vi "Ejercicio 2.4.vi"() -> ()   [LabVIEW 2013]
panel:
  in  "Funcion":T1(ring)
  in  "stop 2":bool
  out "Waveform Graph":dbl[](graph)
  in  "Amplitud":dbl
  in  "Frecuencia":dbl
  in  "Cantidad de muestras":i32=20
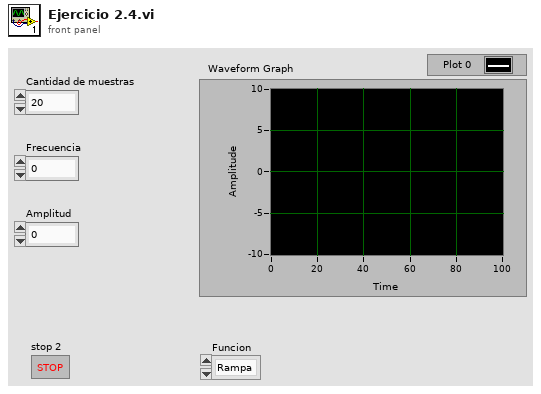
[diagram p1: front panel]
types:
  T1 = enum16{"Rampa", "Seno", "Triangular", "Cuadrado"}
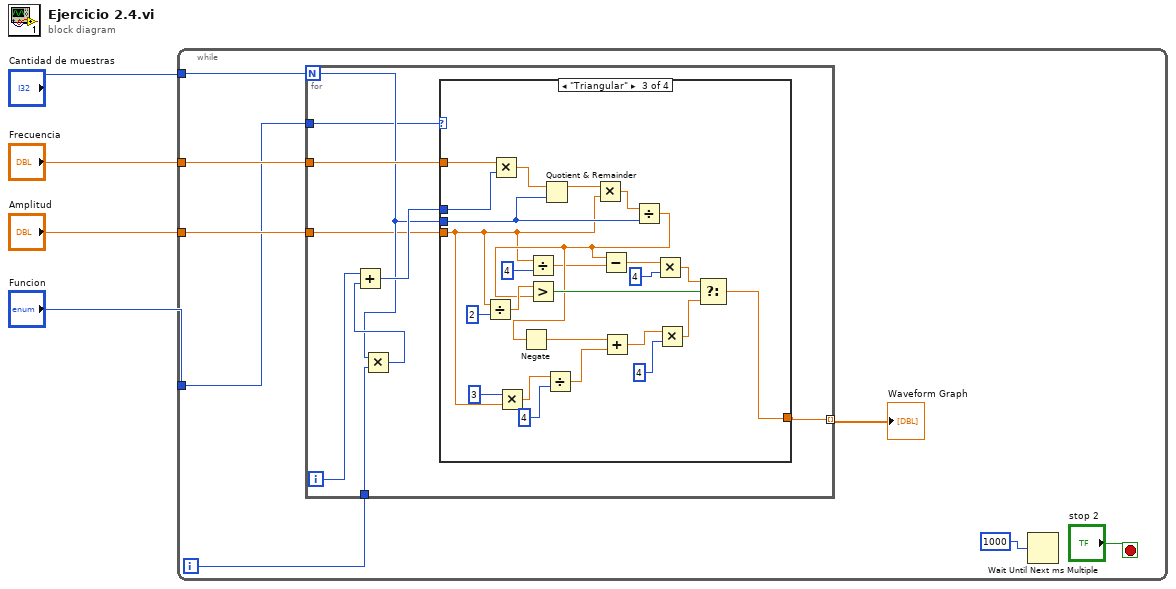
[diagram p0: block diagram]
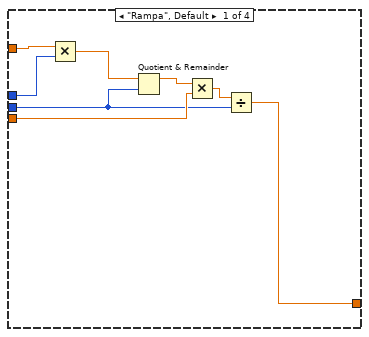
[diagram p2: hidden frame]
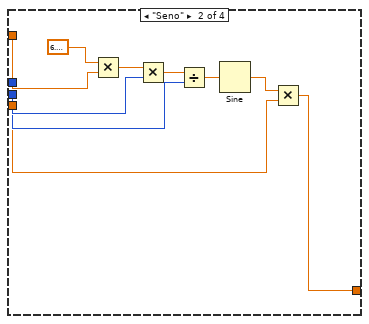
[diagram p3: hidden frame]
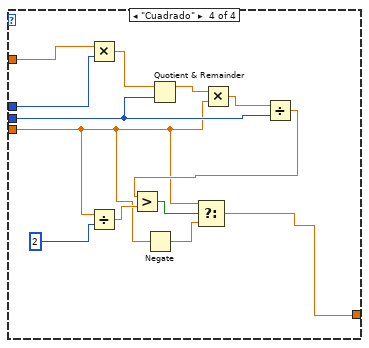
[diagram p4: hidden frame]
diagram:
  n1 = while {
    tunnel: "Cantidad de muestras" -> [w10]
    tunnel: "Frecuencia" -> [w7]
    tunnel: "Amplitud" -> [w9]
    tunnel: "Funcion" -> [w5]
    i -> [w8]
    stop <- "stop 2" stop-if-true
    n2 = for {
      N: w10 -> [w16]
      tunnel: w9 -> [w15]
      tunnel: w8 -> [w19]
      tunnel: w7 -> [w18]
      tunnel: [w14] -> w6 mode=indexing
      tunnel: w5 -> [w13]
      i -> [w21]
      n3 = Multiply(x=w16, y=w19) -> (x*y=w20:i32)
      n4 = Add(x=w21, y=w20) -> (x+y=w17:i32)
      n5 = case shown="\"Triangular\"" w13 {
        tunnel: w18 -> [w29 w38 w61 w74]
        tunnel: w17 -> [w28 w36 w60 w73]
        tunnel: w16 -> [w23 w34 w59 w72]
        tunnel: w15 -> [w25 w31 w45 w66]
        tunnel: [w22 w30 w56 w68] -> w14
        frame "Rampa", Default {
          n6 = Multiply(x=w29, y=w28) -> (x*y=w27:dbl)
          n7 = Quotient & Remainder(x=w27, y=w23) -> (x-y*floor(x/y)=w26:dbl)  [unwired: 1 out]
          n8 = Multiply(x=w26, y=w25) -> (x*y=w24:dbl)
          n9 = Divide(x=w24, y=w23) -> (x/y=w22:dbl)
        }
        frame "Seno" {
          n10 = Multiply(x=6.283185307179586, y=w38) -> (x*y=w37:dbl)
          n11 = Multiply(x=w37, y=w36) -> (x*y=w35:dbl)
          n12 = Divide(x=w35, y=w34) -> (x/y=w33:dbl)
          n13 = Sine(x=w33) -> (sin(x)=w32:dbl)
          n14 = Multiply(x=w32, y=w31) -> (x*y=w30:dbl)
        }
        frame "Triangular" {
          n15 = Divide(x=w45, y=2) -> (x/y=w55:dbl)
          n16 = Multiply(x=w61, y=w60) -> (x*y=w64:dbl)
          n17 = Multiply(x=3, y=w45) -> (x*y=w43:dbl)
          n18 = Divide(x=w45, y=4) -> (x/y=w46:dbl)
          n19 = Quotient & Remainder(x=w64, y=w59) -> (x-y*floor(x/y)=w63:dbl)  [unwired: 1 out]
          n20 = Divide(x=w43, y=4) -> (x/y=w40:dbl)
          n21 = Multiply(x=w63, y=w45) -> (x*y=w62:dbl)
          n22 = Divide(x=w62, y=w59) -> (x/y=w54:dbl)
          n23 = Negate(x=w54) -> (-x=w41:dbl)
          n24 = Greater?(x=w55, y=w54) -> (0:w57:bool)
          n25 = Subtract(x=w54, y=w46) -> (x-y=w53:dbl)
          n26 = Add(x=w41, y=w40) -> (x+y=w49:dbl)
          n27 = Multiply(x=w53, y=4) -> (x*y=w51:dbl)
          n28 = Multiply(x=w49, y=4) -> (x*y=w48:dbl)
          n29 = Select(t=w51, s=w57, f=w48) -> (s? t:f=w56:dbl)
        }
        frame "Cuadrado" {
          n30 = Multiply(x=w74, y=w73) -> (x*y=w75:dbl)
          n31 = Divide(x=w66, y=2) -> (x/y=w69:dbl)
          n32 = Negate(x=w66) -> (-x=w65:dbl)
          n33 = Quotient & Remainder(x=w75, y=w72) -> (x-y*floor(x/y)=w76:dbl)  [unwired: 1 out]
          n34 = Multiply(x=w76, y=w66) -> (x*y=w77:dbl)
          n35 = Divide(x=w77, y=w72) -> (x/y=w71:dbl)
          n36 = Greater?(x=w71, y=w69) -> (0:w67:bool)
          n37 = Select(t=w66, s=w67, f=w65) -> (s? t:f=w68:dbl)
        }
      }
    }
    "Waveform Graph" <- w6
    n38 = Wait Until Next ms Multiple(millisecond multiple=1000) -> ()  [unwired: 1 out]
  }
